vi "write_new_values_to_scope_controls.vi"(0 "Controls Cluster":T5 {"C1 vertical coupling / V" items=["AC", "DC", "Ground"]; "C2 vertical coupling / V" items=["AC", "DC", "Ground"]; "Trigger slope" items=["Positive", "Negative"]}, 7 "Controls References Cluster":T1, 11 "error in (no error)":errorcluster) -> (15 "error out":errorcluster)   [LabVIEW 2023]
uses:
  <instrlib>/niScope/Controls/niScope vertical coupling.ctl
  <instrlib>/niScope/Controls/niScope trigger source.ctl
  <instrlib>/niScope/Controls/niScope trigger slope.ctl
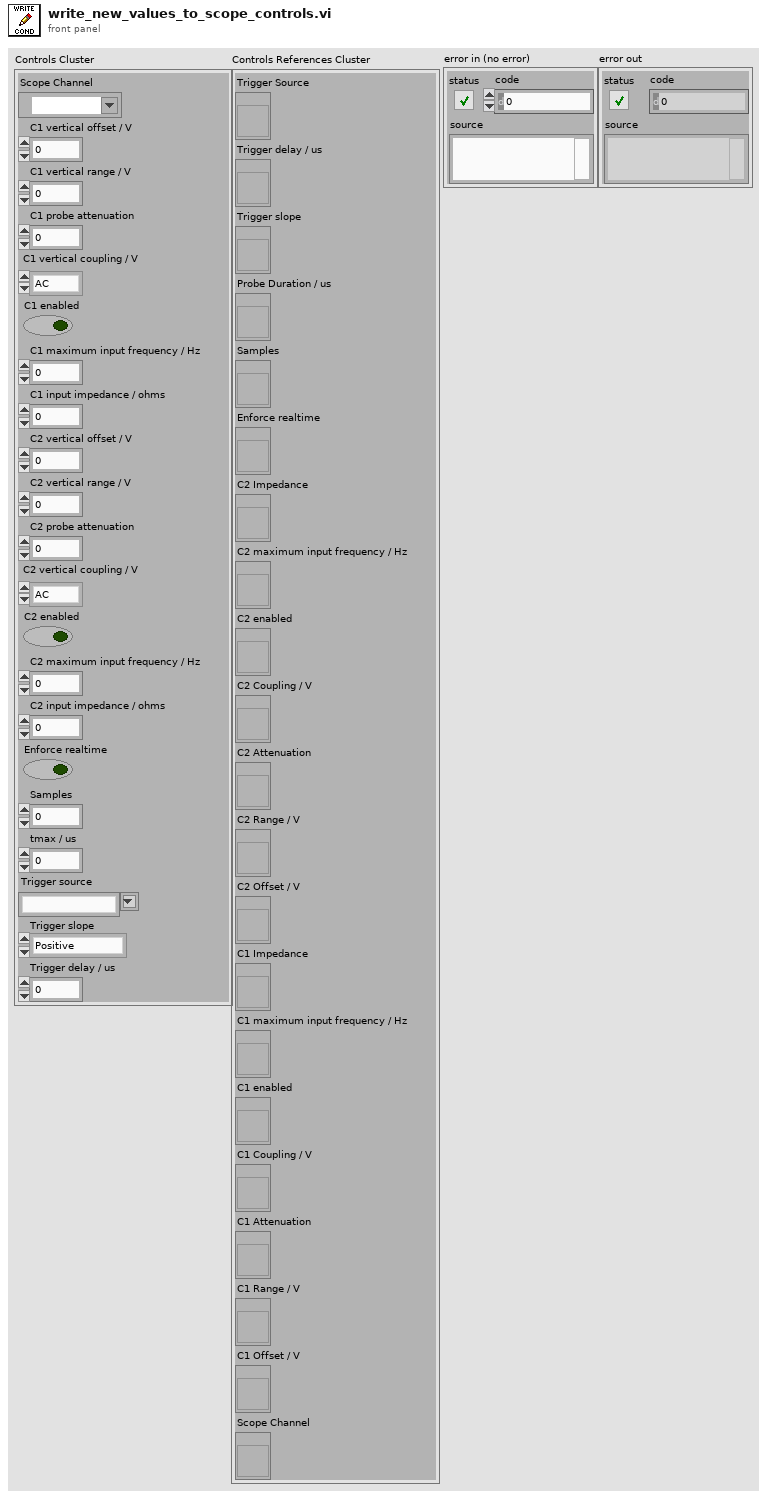
[diagram p1: front panel]
types:
  T1 = cluster{"Trigger Source":refnum<vi>, "Trigger delay / us":refnum<vi>, "Trigger slope":refnum<vi>, "Probe Duration / us":refnum<vi>, "Samples":refnum<vi>, "Enforce realtime":refnum<vi>, "C2 Impedance":refnum<vi>, "C2 maximum input frequency / Hz":refnum<vi>, "C2 enabled":refnum<vi>, "C2 Coupling / V":refnum<vi>, "C2 Attenuation":refnum<vi>, "C2 Range / V":refnum<vi>, "C2 Offset / V":refnum<vi>, "C1 Impedance":refnum<vi>, "C1 maximum input frequency / Hz":refnum<vi>, "C1 enabled":refnum<vi>, "C1 Coupling / V":refnum<vi>, "C1 Attenuation":refnum<vi>, "C1 Range / V":refnum<vi>, "C1 Offset / V":refnum<vi>, "Scope Channel":refnum<vi>}
  T2 = typedef "niScope vertical coupling.ctl" = i32
  T3 = typedef "niScope trigger source.ctl" = string
  T4 = typedef "niScope trigger slope.ctl" = i32
  T5 = cluster{"Scope Channel":refnum<k15>, "C1 vertical offset / V":dbl, "C1 vertical range / V":dbl, "C1 probe attenuation":dbl, "C1 vertical coupling / V":T2, "C1 enabled":bool, "C1 maximum input frequency / Hz":dbl, "C1 input impedance / ohms":u32, "C2 vertical offset / V":dbl, "C2 vertical range / V":dbl, "C2 probe attenuation":dbl, "C2 vertical coupling / V":T2, "C2 enabled":bool, "C2 maximum input frequency / Hz":dbl, "C2 input impedance / ohms":u32, "Enforce realtime":bool, "Samples":i64, "tmax / us ":dbl, "Trigger source":T3, "Trigger slope":T4, "Trigger delay / us":dbl}
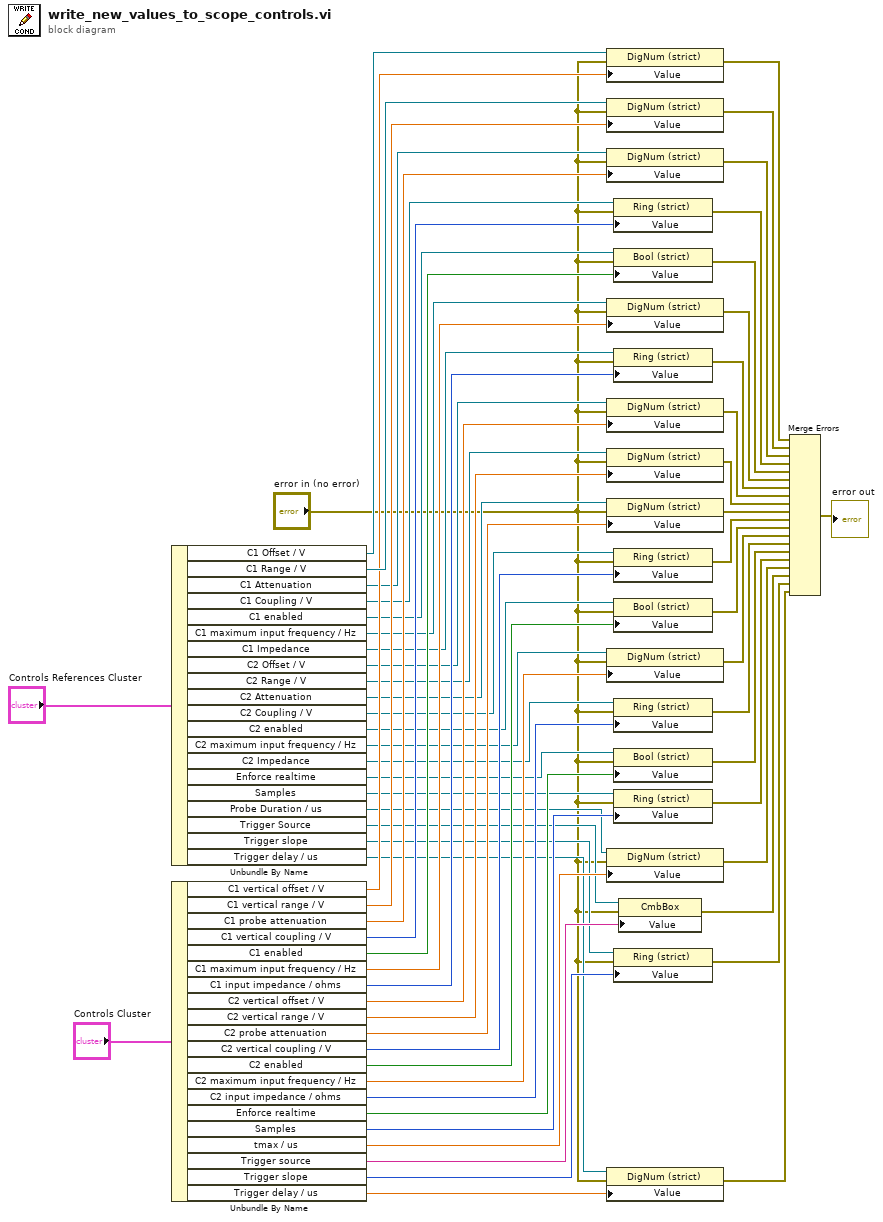
[diagram p0: block diagram]
diagram:
  n1 = Unbundle By Name("Controls References Cluster") -> ("C1 Offset / V"=w60:refnum<vi>, "C1 Range / V"=w59:refnum<vi>, "C1 Attenuation"=w56:refnum<vi>, "C1 Coupling / V"=w52:refnum<vi>, "C1 enabled"=w50:refnum<vi>, "C1 maximum input frequency / Hz"=w48:refnum<vi>, "C1 Impedance"=w42:refnum<vi>, "C2 Offset / V"=w40:refnum<vi>, "C2 Range / V"=w37:refnum<vi>, "C2 Attenuation"=w34:refnum<vi>, "C2 Coupling / V"=w32:refnum<vi>, "C2 enabled"=w28:refnum<vi>, "C2 maximum input frequency / Hz"=w26:refnum<vi>, "C2 Impedance"=w24:refnum<vi>, "Enforce realtime"=w22:refnum<vi>, "Samples"=w20:refnum<vi>, "Probe Duration / us"=w18:refnum<vi>, "Trigger Source"=w16:refnum<vi>, "Trigger slope"=w14:refnum<vi>, "Trigger delay / us"=w12:refnum<vi>)
  n2 = Unbundle By Name("Controls Cluster") -> ("C1 vertical offset / V"=w58:dbl, "C1 vertical range / V"=w57:dbl, "C1 probe attenuation"=w55:dbl, "C1 vertical coupling / V"=w51:T2, "C1 enabled"=w49:bool, "C1 maximum input frequency / Hz"=w47:dbl, "C1 input impedance / ohms"=w41:u32, "C2 vertical offset / V"=w39:dbl, "C2 vertical range / V"=w36:dbl, "C2 probe attenuation"=w33:dbl, "C2 vertical coupling / V"=w31:T2, "C2 enabled"=w27:bool, "C2 maximum input frequency / Hz"=w25:dbl, "C2 input impedance / ohms"=w23:u32, "Enforce realtime"=w21:bool, "Samples"=w19:i64, "tmax / us"=w17:dbl, "Trigger source"=w15:T3, "Trigger slope"=w13:T4, "Trigger delay / us"=w11:dbl)
  n3 = property class="DigNum (strict)"(reference=w60, error in="error in (no error)", "Value"=w58) -> (error out=w63:errorcluster)  [unwired: 1 out]
  n4 = property class="DigNum (strict)"(reference=w59, error in="error in (no error)", "Value"=w57) -> (error out=w54:errorcluster)  [unwired: 1 out]
  n5 = property class="DigNum (strict)"(reference=w56, error in="error in (no error)", "Value"=w55) -> (error out=w53:errorcluster)  [unwired: 1 out]
  n6 = property class="DigNum (strict)"(reference=w48, error in="error in (no error)", "Value"=w47) -> (error out=w44:errorcluster)  [unwired: 1 out]
  n7 = property class="DigNum (strict)"(reference=w40, error in="error in (no error)", "Value"=w39) -> (error out=w38:errorcluster)  [unwired: 1 out]
  n8 = property class="DigNum (strict)"(reference=w37, error in="error in (no error)", "Value"=w36) -> (error out=w35:errorcluster)  [unwired: 1 out]
  n9 = property class="DigNum (strict)"(reference=w34, error in="error in (no error)", "Value"=w33) -> (error out=w30:errorcluster)  [unwired: 1 out]
  n10 = property class="DigNum (strict)"(reference=w26, error in="error in (no error)", "Value"=w25) -> (error out=w9:errorcluster)  [unwired: 1 out]
  n11 = property class="DigNum (strict)"(reference=w18, error in="error in (no error)", "Value"=w17) -> (error out=w5:errorcluster)  [unwired: 1 out]
  n12 = property class="DigNum (strict)"(reference=w12, error in="error in (no error)", "Value"=w11) -> (error out=w2:errorcluster)  [unwired: 1 out]
  n13 = property class="Ring (strict)"(reference=w52, error in="error in (no error)", "Value"=w51) -> (error out=w46:errorcluster)  [unwired: 1 out]
  n14 = property class="Bool (strict)"(reference=w50, error in="error in (no error)", "Value"=w49) -> (error out=w45:errorcluster)  [unwired: 1 out]
  n15 = property class="Ring (strict)"(reference=w42, error in="error in (no error)", "Value"=w41) -> (error out=w43:errorcluster)  [unwired: 1 out]
  n16 = property class="Ring (strict)"(reference=w32, error in="error in (no error)", "Value"=w31) -> (error out=w29:errorcluster)  [unwired: 1 out]
  n17 = property class="Bool (strict)"(reference=w28, error in="error in (no error)", "Value"=w27) -> (error out=w10:errorcluster)  [unwired: 1 out]
  n18 = property class="Ring (strict)"(reference=w24, error in="error in (no error)", "Value"=w23) -> (error out=w8:errorcluster)  [unwired: 1 out]
  n19 = property class="Bool (strict)"(reference=w22, error in="error in (no error)", "Value"=w21) -> (error out=w7:errorcluster)  [unwired: 1 out]
  n20 = property class="Ring (strict)"(reference=w20, error in="error in (no error)", "Value"=w19) -> (error out=w6:errorcluster)  [unwired: 1 out]
  n21 = property class="Ring (strict)"(reference=w14, error in="error in (no error)", "Value"=w13) -> (error out=w3:errorcluster)  [unwired: 1 out]
  n22 = property class="CmbBox"(reference=w16, error in="error in (no error)", "Value"=w15) -> (error out=w4:errorcluster)  [unwired: 1 out]
  n23 = Merge Errors(w63, w54, w53, w46, w45, w44, w43, w38, w35, w30, w29, w10, w9, w8, w7, w6, w5, w4, w3, w2) -> (→"error out":errorcluster)
